vi "WPI_CAN_PDPSend.vi"(11 "Power Distribution Panel (0)":u8) -> (3 "Power Distribution Panel Out":u8)   [LabVIEW 2017]
uses:
  <vilib>/Rock Robotics/WPI/CAN/PDP/WPI_CAN_PDPMessageIDs.ctl
  <vilib>/Rock Robotics/WPI/CAN/PDP/WPI_CAN_PDPGlobalOps.ctl
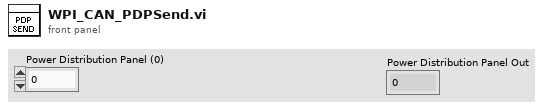
[diagram p1: front panel]
types:
  T1 = typedef "WPI_CAN_PDPGlobalOps.ctl" = enum16{"Write After Receive 0-5", "Write After Receive 6-11", "Write After Receive 12-15", "Write After Receive Energy", "Get All", "Get Commands", "Write Clear Sticky Faults Command", "Write Reset Energy Command", "Write Tare Currents Command", "Write Error", "Write After Receive Faults"}
  T2 = typedef "WPI_CAN_PDPMessageIDs.ctl" = u32
  T3 = typedef "WPI_CAN_PDPCommands.ctl" = cluster{"Tare Currents":bool, "Reset Energy":bool, "Clear Sticky Faults":bool}
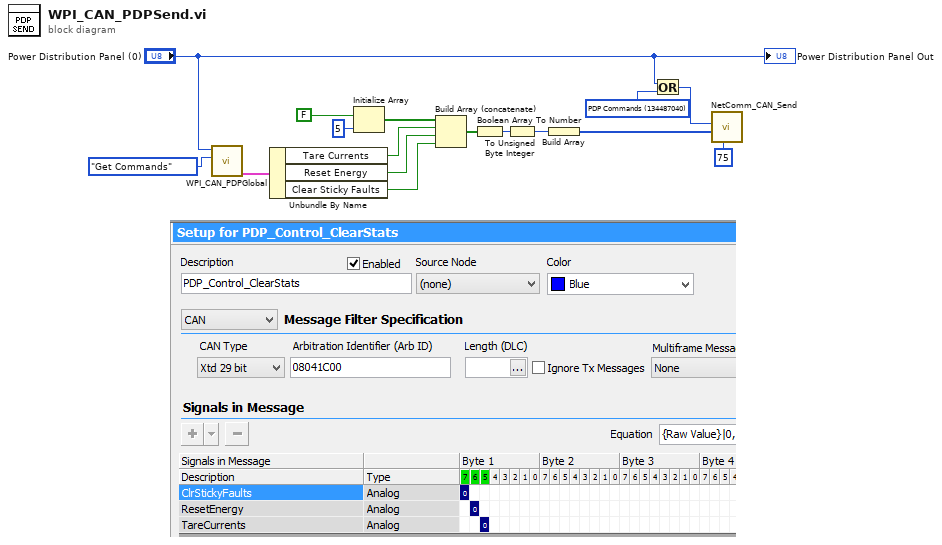
[diagram p0: block diagram]
diagram:
  w16 = T2 134487040 items=["PDP Status 0-5"=134484992, "PDP Status 6-11"=134485056, "PDP Status 12-15"=134485120, "PDP Faults & Stats"=134485184, "PDP Energy"=134485824, "PDP Commands"=134487040, "PDP Update Event"=134487168, "PDP Update Robot State"=134487104] ("PDP Message IDs")
  n1 = call <vilib>:"WPI_CAN_PDPGlobal.vi"("Operation"=WPI_CAN_PDPGlobalOps."Get Commands", "Power Distribution Panel (0)"="Power Distribution Panel (0)") -> ("Commands"=w12:T3)  [unwired: 7 in, 2 out]
  n2 = Unbundle By Name(w12) -> ("Tare Currents"=w8:bool, "Reset Energy"=w7:bool, "Clear Sticky Faults"=w6:bool)
  n3 = Initialize Array(FALSE, 5 ("dimension size")) -> (w9:bool[])
  n4 = Build Array (concatenate)(w9, w8, w7, w6) -> (w5:bool[])
  n5 = Boolean Array To Number(Boolean array=w5) -> (number=w4:u32)
  n6 = To Unsigned Byte Integer(number=w4) -> (unsigned 8bit integer=w3:u8)
  n7 = Build Array(w3) -> (w2:u8[])
  n8 = Or(x="Power Distribution Panel (0)", y=w16) -> (x .or. y?=w15:T2)
  n9 = call <vilib>:"NetComm_CAN_Send.vi"("Period (ms)"=75, "Data"=w2, "Message ID"=w15) -> ()  [unwired: 8 in, 1 out]
  "Power Distribution Panel Out" <- "Power Distribution Panel (0)"
